vi "Func Processor for K-Laws-16032016.vi"(8 "Math Expressions In":string[](array[string]), 9 "Fn Arg Cnt":string[](array[string]), 10 "Functions Definition":string[][](table), 11 "Total Function Definitions":i32) -> (3 "Math Expressions Out":string[](array[string]))   [LabVIEW 2014]
panel:
  out "Fn Variables":string[](array[string])
  out "Actual Variable":string[](array[string])
  out "Function Formula":string
  out "Fn-Math":string[](array[string])
  out "Fn Name":string[](array[string])
  # "External Inputs"
  # "Intermediate variables"
  # "Outputs"
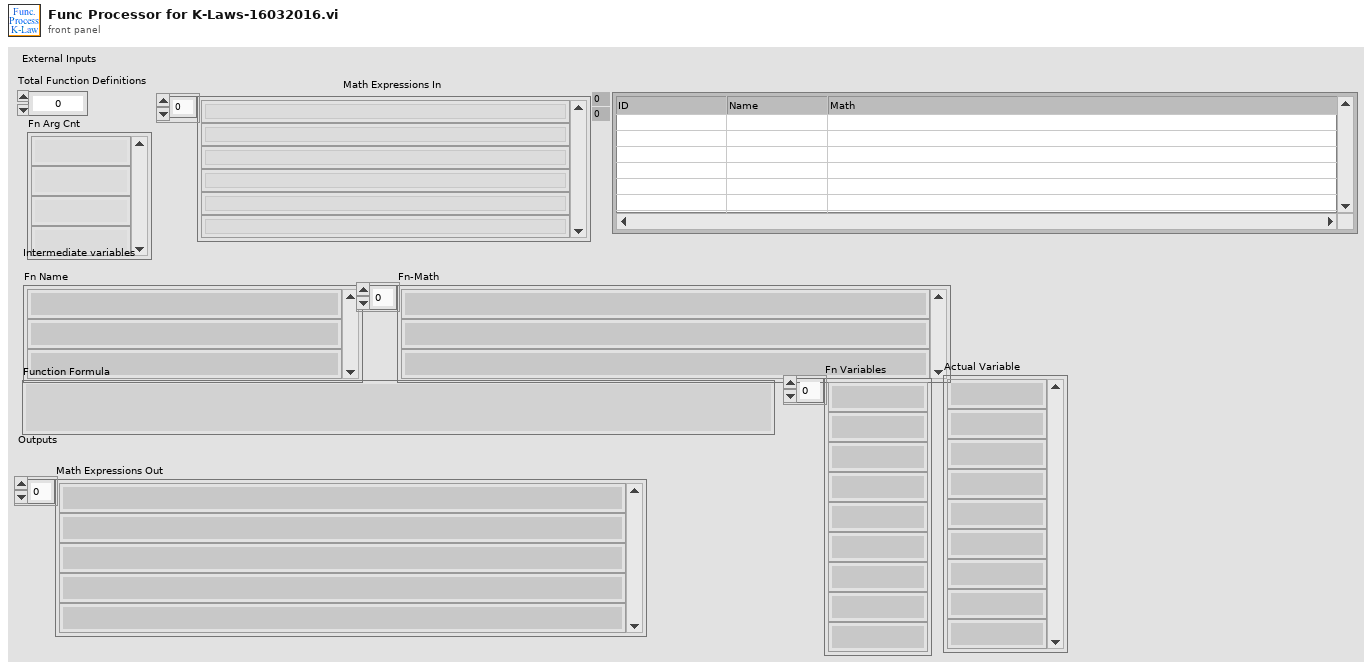
[diagram p1: front panel]
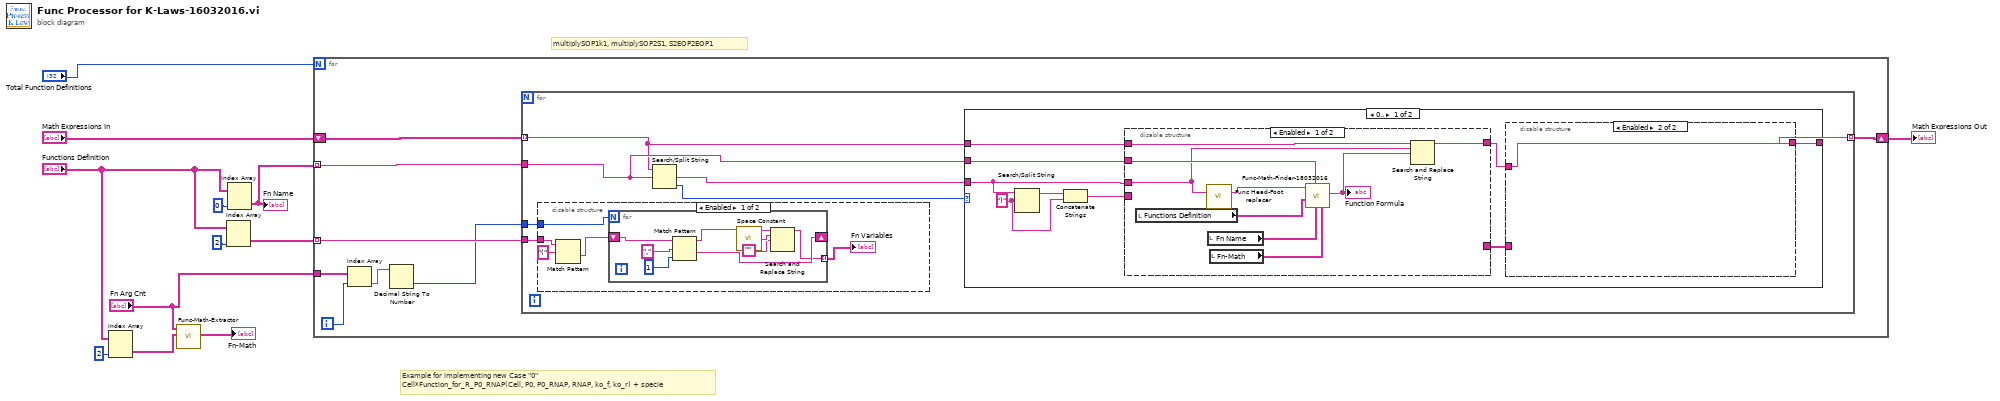
[diagram p0: block diagram]
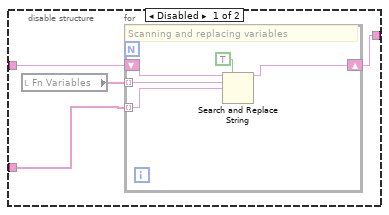
[diagram p3: hidden frame]
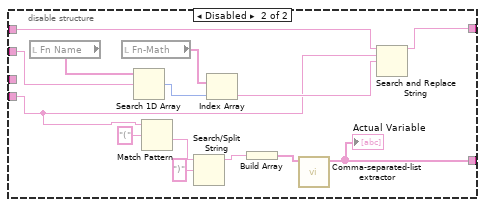
[diagram p4: hidden frame]
diagram:
  # "Example for implementing new Case \"0\" \nCell*Function_for_R_P0_RNAP(Cell, P0, P0_RNAP, RNAP, ko_f, ko_r) + specie"
  # "multiplySOP1k1, multiplySOP2S1, S2EOP2EOP1"
  n1 = Index Array(array="Functions Definition", index (col)=2 ("disabled index (col)")) -> (element=w7:string[])  [unwired: 1 in]
  n2 = call "Func-Math-Extractor.vi"("Fn Math"=w7, "Fn Arg Cnt"="Fn Arg Cnt") -> ("Fn-Math"=→"Fn-Math":string[])  [unwired: 9 in]
  n3 = Index Array(array="Functions Definition", index (col)=2 ("disabled index (col)")) -> (element=w2:string[])  [unwired: 1 in]
  n4 = Index Array(array="Functions Definition", index (col)=0 ("disabled index (col)")) -> (element=w9:string[])  [unwired: 1 in]
  "Fn Name" <- w9
  n5 = for {
    N: "Total Function Definitions" -> [_]
    tunnel: w9 -> [w19] mode=indexing
    shift-right: [w18] -> w5
    shift-left: "Math Expressions In" -> [w20]
    tunnel: w2 -> [w17] mode=indexing
    tunnel: "Fn Arg Cnt" -> [w14]
    i -> [w15]
    n6 = Index Array(array=w14, index=w15) -> (element=w16:string)
    n7 = Decimal String To Number(string=w16) -> (number=w13:i32)  [unwired: 2 in, 1 out]
    n8 = for {
      tunnel: w20 -> [w24] mode=indexing
      tunnel: w19 -> [w26]
      tunnel: [w23] -> w18 mode=indexing
      tunnel: w17 -> [w21]
      tunnel: w13 -> [w22]
      n9 = disable-structure shown="Enabled" {
        disable-tunnel: w21 -> [w31 _]
        disable-tunnel: w22 -> [w28 _]
        frame Enabled {
          n10 = Match Pattern(string=w31, regular expression="(") -> (after substring=w30:string)  [unwired: 1 in, 3 out]
          n11 = for {
            N: w28 -> [_]
            shift-right: [w37] -> _
            shift-left: w30 -> [w40]
            tunnel: [w33] -> w29 mode=indexing
            n12 = Match Pattern(string=w40, regular expression="," ("search string/char (-)"), offset (0)=1) -> (before substring=w34:string, after substring=w37:string)  [unwired: 2 out]
            n13 = call <vilib>:"Space Constant.vi"() -> ("String"=w36:string)
            n14 = Search and Replace String(input string=w34, search string=w36, replace string="") -> (result string=w33:string)  [unwired: 5 in, 3 out]
          }
          "Fn Variables" <- w29
        }
        frame Disabled {
        }
      }
      n15 = Search/Split String(string=w24, search string/char (-)=w26) -> (match + rest of string=w27:string, offset of match=w25:i32)  [unwired: 1 in, 1 out]
      n16 = case shown="0.." w25 {
        tunnel: w27 -> [w41 _]
        tunnel: w26 -> [w49 _]
        tunnel: w24 -> [w48 w83]
        tunnel: [w42 w83] -> w23
        frame 0.. {
          w46 = ")" ("search string/char (-)")
          n17 = Search/Split String(string=w41, search string/char (-)=w46) -> (substring before match=w47:string)  [unwired: 1 in, 2 out]
          n18 = Concatenate Strings(w47, w46) -> (w45:string)
          n19 = disable-structure shown="Enabled" {
            disable-tunnel: w49 -> [w67 w76]
            disable-tunnel: w48 -> [w64 w79]
            disable-tunnel: [w62 w77] -> w44
            disable-tunnel: w45 -> [_ w70]
            disable-tunnel: [_ w69] -> w43
            disable-tunnel: w41 -> [w61 _]
            frame Enabled {
              n20 = local read "Functions Definition"() -> (w60:string[][])
              n21 = call "Func Head-Foot replacer.vi"("Function in"=w61) -> ("Function in Out"=w68:string)  [unwired: 12 in, 2 out]
              n22 = local read "Fn Name"() -> (w66:string[])
              n23 = local read "Fn-Math"() -> (w65:string[])
              n24 = call "Func-Math-Finder-18032016.vi"("All Fn-Math"=w65, "All Fn Name"=w66, "Func Name"=w67, "Functions Definition"=w60, "Get Tagged String"=w68) -> ("Expression"=w63:string)  [unwired: 4 in, 2 out]
              "Function Formula" <- w63
              n25 = Search and Replace String(input string=w64, search string=w61, replace string=w63) -> (result string=w62:string)  [unwired: 5 in, 3 out]
            }
            frame Disabled {
              n26 = local read "Fn Name"() -> (w82:string[])
              n27 = local read "Fn-Math"() -> (w81:string[])
              n28 = Search 1D Array(1D array=w82, element=w76) -> (index of element=w80:i32)  [unwired: 1 in]
              n29 = Match Pattern(string=w70, regular expression="(" ("search string/char (-)")) -> (after substring=w73:string)  [unwired: 1 in, 3 out]
              n30 = Search/Split String(string=w73, search string/char (-)=")") -> (substring before match=w74:string)  [unwired: 1 in, 2 out]
              n31 = Index Array(array=w81, index=w80) -> (element=w78:string)
              n32 = Build Array(w74) -> (w75:string[])
              n33 = call "Comma-separated-list extractor.vi"("In_list"=w75) -> ("List_Out"=w69:string[])  [unwired: 6 in, 1 out]
              "Actual Variable" <- w69
              n34 = Search and Replace String(input string=w79, search string=w70, replace string=w78) -> (result string=w77:string)  [unwired: 5 in, 3 out]
            }
          }
          n35 = disable-structure shown="Enabled" {
            disable-tunnel: w44 -> [w52 w59]
            disable-tunnel: w43 -> [w51 _]
            disable-tunnel: [w50 w59] -> w42
            frame Disabled {
              n36 = local read "Fn Variables"() -> (w53:string[])
              n37 = for {
                tunnel: w53 -> [w57] mode=indexing
                tunnel: w51 -> [w56] mode=indexing
                shift-right: [w54] -> w50
                shift-left: w52 -> [w58]
                # "Scanning and replacing variables"
                n38 = Search and Replace String(replace all?=TRUE ("replace all? (F)"), input string=w58, search string=w57, replace string=w56) -> (result string=w54:string)  [unwired: 4 in, 3 out]
              }
            }
            frame Enabled {
            }
          }
        }
        frame -1, Default {
        }
      }
    }
  }
  "Math Expressions Out" <- w5
